vi "STAT 2 Stroker Decode Analog Data.vi"(0 "Received(T)":bool=TRUE, 7 "Controller SATT 2":T2 {"Tension Sub 2"."sys register" format="%04x"; "Tension Sub 1"."sys register" format="%04x"; "PSU"."sys register" format="%04x"; "solonoid"."valve status" format="%02x"; "solonoid"."sys register" format="%04x"; "pressure 2"."sys register" format="%04x"; "pressure 1"."sys register" format="%04x"; "Controller local"."High G monitoring" format="%02x"; "Controller local"."NA" format="%02x"; "Controller local"."GPIO values" format="%02x"; "Controller local"."Relay status" format="%02x"; "Controller local"."sys register" format="%04x"}, 11 "error in (no error)":errorcluster) -> (6 "Tool analog value":dbl[](array[numeric]), 8 "Analog for digital calc":T1, 10 "Tool analog index":u16[](array[numeric]), 14 "Solenoid position":dbl, 15 "error out":errorcluster)   [LabVIEW 2011]
uses:
  High level/Variable List Stroker Analog.ctl
  Analog values for digital calculations.ctl
  LEINmaster/Nodes/Controller local stat2.ctl
  LEINmaster/Nodes/pressure stat2.ctl
  LEINmaster/Nodes/solonoid stat2.ctl
  Stat def/Stroker system stat2.ctl
  LEINmaster/Nodes/PSU stat2.ctl
  LEINmaster/Nodes/tensionsub stat2.ctl
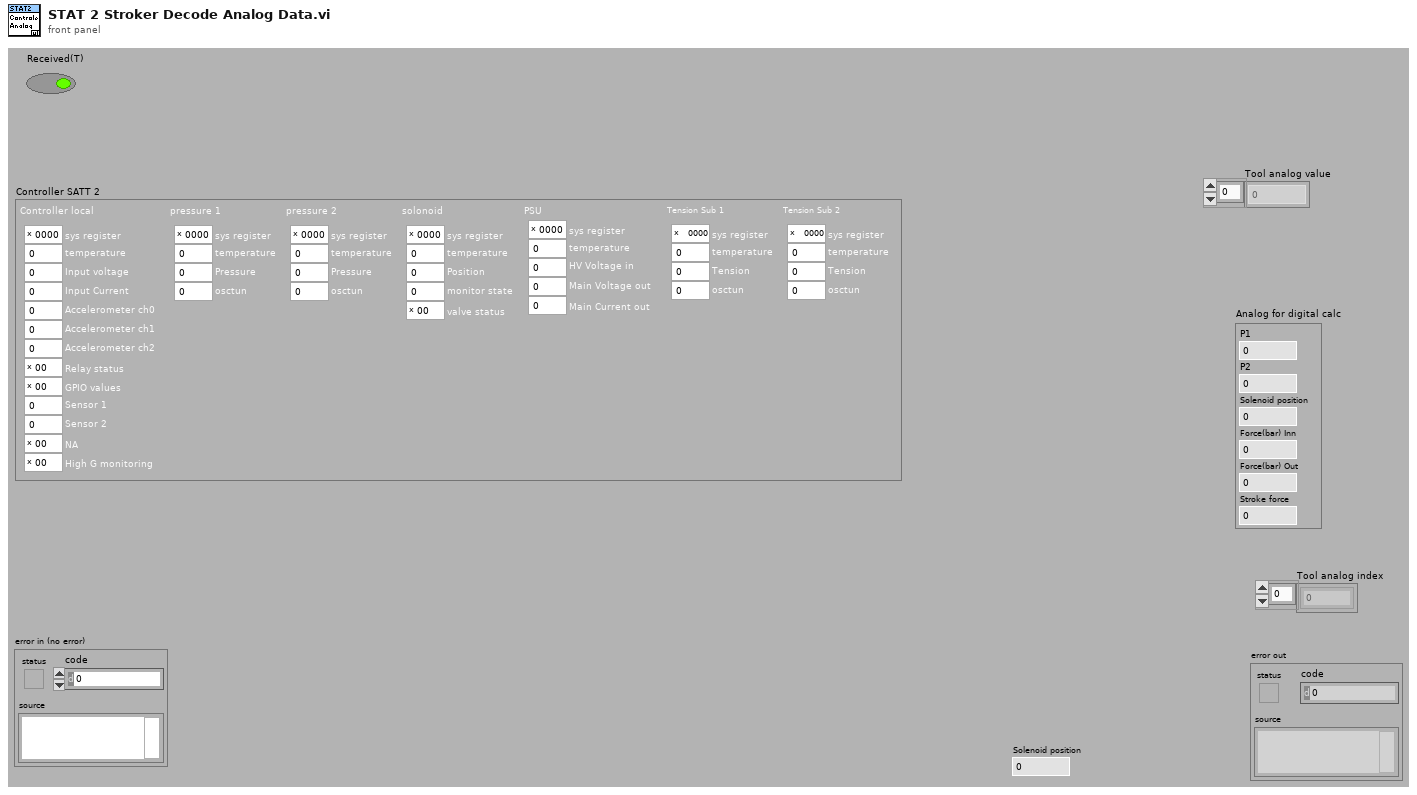
[diagram p1: front panel]
types:
  T1 = typedef "Analog values for digital calculations.ctl" = cluster{"P1":dbl, "P2":dbl, "Solenoid position":dbl, "Force(bar) Inn":dbl, "Force(bar) Out":dbl, "Stroke force":dbl}
  T2 = typedef "Stroker system stat2.ctl" = cluster{"Controller local":T3, "pressure 1":T4, "pressure 2":T4, "solonoid":T5, "PSU":T6, "Tension Sub 1":T7, "Tension Sub 2":T7}
  T3 = typedef "Controller local stat2.ctl" = cluster{"sys register":u16, "temperature":u16, "Input voltage":u16, "Input Current":u16, "Accelerometer ch0":u16, "Accelerometer ch1":u16, "Accelerometer ch2":u16, "Relay status":u8, "GPIO values":u8, "Sensor 1":i32, "Sensor 2":i32, "NA":u8, "High G monitoring":u8}
  T4 = typedef "pressure stat2.ctl" = cluster{"sys register":u16, "temperature":u16, "Pressure":u16, "osctun":u8}
  T5 = typedef "solonoid stat2.ctl" = cluster{"sys register":u16, "temperature":u16, "Position":i16, "monitor state":u8, "valve status":u8}
  T6 = typedef "PSU stat2.ctl" = cluster{"sys register":u16, "temperature":u16, "HV Voltage in":u16, "Main Voltage out":u16, "Main Current out":u16}
  T7 = typedef "tensionsub stat2.ctl" = cluster{"sys register":u16, "temperature":u16, "Tension":i16, "osctun":u8}
  T8 = typedef "Variable List Stroker Analog.ctl" = enum16{"Tool max Temperature", "Solenoid Temp", "Tool supply Voltage", "Tool (Controller) Current", "Tool Acceleration X", "Tool Acceleration Y", "Tool Acceleration Z", "Controller Temp", "Tool Acceleration Sum", "Tool Inclination", "Tool Rotation", "Tool Stroke Extension", "Tool GP Sensor 1", "Tool GP Sensor 2", "Tool (Pressure 1) Temp", "Tool Pressure 1", "Tool (Pressure 2) Temp", "Tool Pressure 2", "Do not use (SIF)", "Do not use (SOF)", "Stroke Force", "PSU Temp", "Head Voltage", "PSU Main Voltage out", "PSU Main Current out", "Upper Tension Sub Temp", "Tool Upper Tension Sub", "Lower Tension Sub Temp", "Tool Lower Tension Sub"}
  T9 = typedef "Options  All pages and custom.ctl" = cluster{"P 1 (App)":T10, "P 2":T11, "P 3":T12, "P 4":T14, "P 5":T18, "P 6 (Err)":T19, "P 7 (Expert)":T20, "C 1":T22, "C 2":T23}
  T10 = typedef "Options Page 1 (App).ctl" = cluster{"Result files":path, "PCP Interface":string, "Stroker Interface":string, "Tractor Interface":string, "Audible Alarm":bool, "Force alarm on Technical":bool, "Force alarm on HH":bool, "Force alarm on LL":bool, "Force alarm on H":bool, "Force alarm on L":bool}
  T11 = typedef "Options Page 2.ctl" = cluster{"Solenoid & Relay latching time":u16, "Tractor relay 1":dbl, "Tractor relay 2":dbl, "Tractor Solenoid limit":dbl}
  T12 = typedef "Options Page 3.ctl" = cluster{"Min resistance":dbl, "Max resistance":dbl, "PCP/PSU range":T13, "Max voltage jump":dbl, "Maximum resistance change":dbl, "Start Telemetry Voltage":dbl, "Start Telemetry Timeout":dbl, "Start Motor Voltage":dbl, "Stop Motor Voltage":dbl, "Pass Mode Warning Voltage":dbl, "Samples to average":i32}
  T13 = typedef "PCP type List.ctl" = enum16{"0 - 350V", "0 - 450V", "0 - 600V"}
  T14 = typedef "Options Page 4.ctl" = cluster{"Solenoid & Relay latching time":u16, "Stroker relay 1":dbl, "Stroker Relay 2":dbl, "Stroker Solenoid limit":dbl, "Force det.":T15, "Stroke force lim.":dbl, "Pressure SLIPS":dbl, "Tacometer puls":dbl, "Relay Voltage Limit":dbl, "Default anchor behavior":T16, "Default stroker behavior":T17, "Default stroker force limit (tonne)":dbl}
  T15 = typedef "Stroke force selector.ctl" = enum16{"Stroke in = node 1", "Strok out = node 1"}
  T16 = typedef "Default anchor behavior.ctl" = enum16{"Do nothing", "Set Anchor", "Release Anchor"}
  T17 = typedef "Default stroker behavior.ctl" = enum16{"Do nothing", "Stop", "Go Out", "Go In"}
  T18 = typedef "Options Page 5.ctl" = cluster{"Solenoid & Relay latching time":u16, "Driller relay 1":dbl, "Driller Relay 2":dbl, "Driller  Solenoid limit":dbl}
  T19 = typedef "Options Page 6 (Err).ctl" = cluster{"Error and event files":path}
  T20 = typedef "Options Page 7 (Expert).ctl" = cluster{"Show Debug":bool, "Log debug messages":bool, "Aditional debug messages":bool, "enumCANCOM":bool, "AutoLogOn":bool, "Buffer size":i32, "Modem sim":T21, "Modem baud":u16, "Upd regular data":bool, "Show Simulator":bool}
  T21 = typedef "Modem simulation setup.ctl" = cluster{"Modem dealay sim":bool, "Sim baud Tx":u16, "Bit Error fraction Tx":dbl, "Sim baud Rx":u16, "Bit Error fraction Rx":dbl}
  T22 = typedef "Options Custom 1.ctl" = cluster{"Placeholder":bool}
  T23 = typedef "Options Custom 2.ctl" = cluster{"Placeholder":bool}
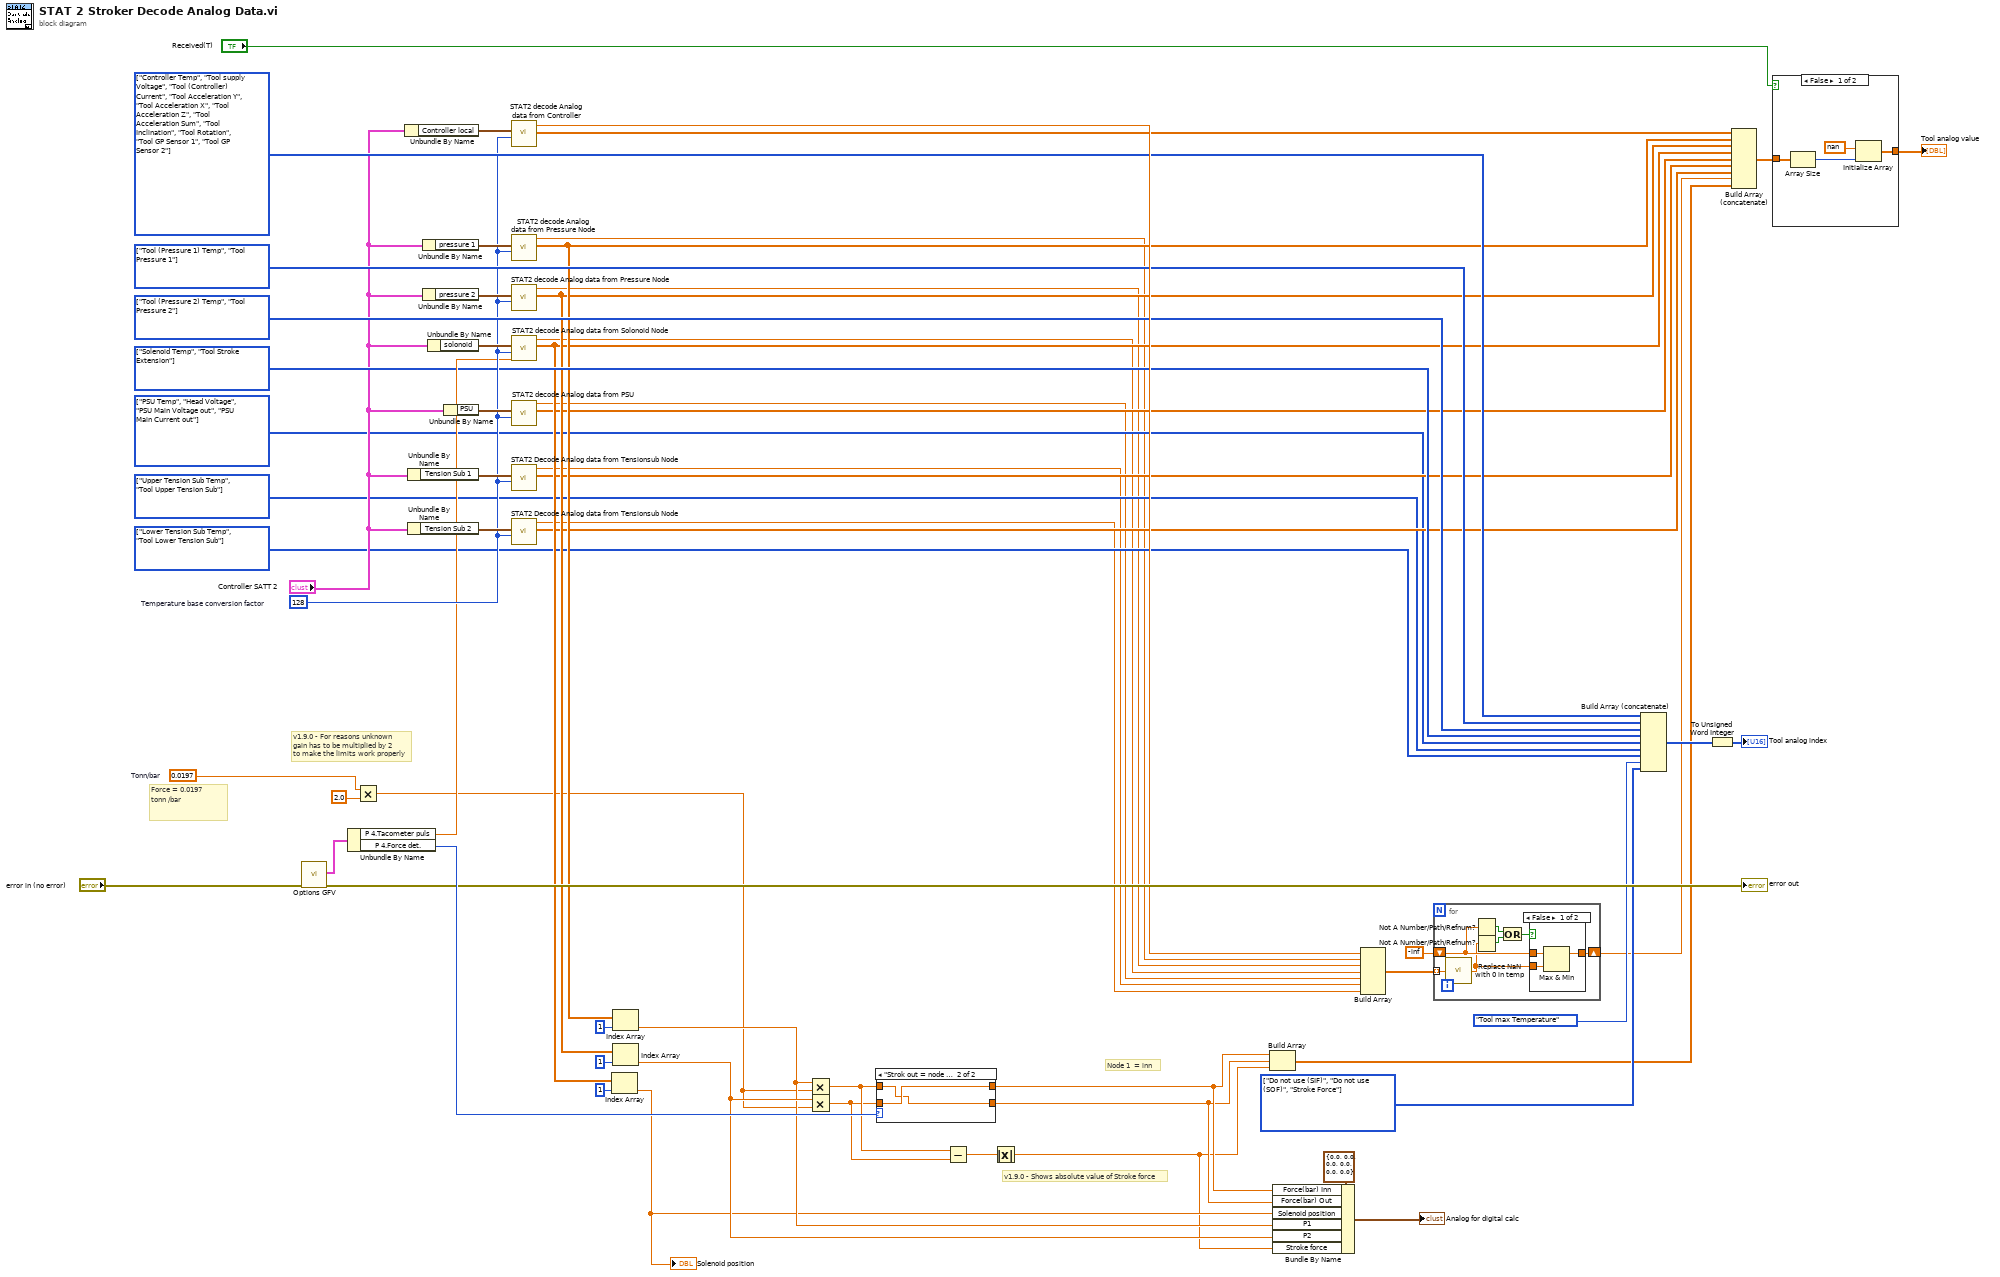
[diagram p0: block diagram]
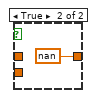
[diagram p3: hidden frame]
diagram:
  w11 = T8[] [enum."Lower Tension Sub Temp", enum."Tool Lower Tension Sub"] items=["Tool max Temperature", "Solenoid Temp", "Tool supply Voltage", "Tool (Controller) Current", "Tool Acceleration X", "Tool Acceleration Y", "Tool Acceleration Z", "Controller Temp", "Tool Acceleration Sum", "Tool Inclination", "Tool Rotation", "Tool Stroke Extension", "Tool GP Sensor 1", "Tool GP Sensor 2", "Tool (Pressure 1) Temp", "Tool Pressure 1", "Tool (Pressure 2) Temp", "Tool Pressure 2", "Do not use (SIF)", "Do not use (SOF)", "Stroke Force", "PSU Temp", "Head Voltage", "PSU Main Voltage out", "PSU Main Current out", "Upper Tension Sub Temp", "Tool Upper Tension Sub", "Lower Tension Sub Temp", "Tool Lower Tension Sub"] ("array")
  w12 = T8[] [enum."Upper Tension Sub Temp", enum."Tool Upper Tension Sub"] items=["Tool max Temperature", "Solenoid Temp", "Tool supply Voltage", "Tool (Controller) Current", "Tool Acceleration X", "Tool Acceleration Y", "Tool Acceleration Z", "Controller Temp", "Tool Acceleration Sum", "Tool Inclination", "Tool Rotation", "Tool Stroke Extension", "Tool GP Sensor 1", "Tool GP Sensor 2", "Tool (Pressure 1) Temp", "Tool Pressure 1", "Tool (Pressure 2) Temp", "Tool Pressure 2", "Do not use (SIF)", "Do not use (SOF)", "Stroke Force", "PSU Temp", "Head Voltage", "PSU Main Voltage out", "PSU Main Current out", "Upper Tension Sub Temp", "Tool Upper Tension Sub", "Lower Tension Sub Temp", "Tool Lower Tension Sub"] ("array")
  w13 = T8[] [enum."PSU Temp", enum."Head Voltage", enum."PSU Main Voltage out", enum."PSU Main Current out"] items=["Tool max Temperature", "Solenoid Temp", "Tool supply Voltage", "Tool (Controller) Current", "Tool Acceleration X", "Tool Acceleration Y", "Tool Acceleration Z", "Controller Temp", "Tool Acceleration Sum", "Tool Inclination", "Tool Rotation", "Tool Stroke Extension", "Tool GP Sensor 1", "Tool GP Sensor 2", "Tool (Pressure 1) Temp", "Tool Pressure 1", "Tool (Pressure 2) Temp", "Tool Pressure 2", "Do not use (SIF)", "Do not use (SOF)", "Stroke Force", "PSU Temp", "Head Voltage", "PSU Main Voltage out", "PSU Main Current out", "Upper Tension Sub Temp", "Tool Upper Tension Sub", "Lower Tension Sub Temp", "Tool Lower Tension Sub"]
  w24 = T8[] [enum."Solenoid Temp", enum."Tool Stroke Extension"] items=["Tool max Temperature", "Solenoid Temp", "Tool supply Voltage", "Tool (Controller) Current", "Tool Acceleration X", "Tool Acceleration Y", "Tool Acceleration Z", "Controller Temp", "Tool Acceleration Sum", "Tool Inclination", "Tool Rotation", "Tool Stroke Extension", "Tool GP Sensor 1", "Tool GP Sensor 2", "Tool (Pressure 1) Temp", "Tool Pressure 1", "Tool (Pressure 2) Temp", "Tool Pressure 2", "Do not use (SIF)", "Do not use (SOF)", "Stroke Force", "PSU Temp", "Head Voltage", "PSU Main Voltage out", "PSU Main Current out", "Upper Tension Sub Temp", "Tool Upper Tension Sub", "Lower Tension Sub Temp", "Tool Lower Tension Sub"]
  w30 = T8[] [enum."Tool (Pressure 2) Temp", enum."Tool Pressure 2"] items=["Tool max Temperature", "Solenoid Temp", "Tool supply Voltage", "Tool (Controller) Current", "Tool Acceleration X", "Tool Acceleration Y", "Tool Acceleration Z", "Controller Temp", "Tool Acceleration Sum", "Tool Inclination", "Tool Rotation", "Tool Stroke Extension", "Tool GP Sensor 1", "Tool GP Sensor 2", "Tool (Pressure 1) Temp", "Tool Pressure 1", "Tool (Pressure 2) Temp", "Tool Pressure 2", "Do not use (SIF)", "Do not use (SOF)", "Stroke Force", "PSU Temp", "Head Voltage", "PSU Main Voltage out", "PSU Main Current out", "Upper Tension Sub Temp", "Tool Upper Tension Sub", "Lower Tension Sub Temp", "Tool Lower Tension Sub"]
  w31 = T8[] [enum."Tool (Pressure 1) Temp", enum."Tool Pressure 1"] items=["Tool max Temperature", "Solenoid Temp", "Tool supply Voltage", "Tool (Controller) Current", "Tool Acceleration X", "Tool Acceleration Y", "Tool Acceleration Z", "Controller Temp", "Tool Acceleration Sum", "Tool Inclination", "Tool Rotation", "Tool Stroke Extension", "Tool GP Sensor 1", "Tool GP Sensor 2", "Tool (Pressure 1) Temp", "Tool Pressure 1", "Tool (Pressure 2) Temp", "Tool Pressure 2", "Do not use (SIF)", "Do not use (SOF)", "Stroke Force", "PSU Temp", "Head Voltage", "PSU Main Voltage out", "PSU Main Current out", "Upper Tension Sub Temp", "Tool Upper Tension Sub", "Lower Tension Sub Temp", "Tool Lower Tension Sub"]
  w32 = T8[] [enum."Controller Temp", enum."Tool supply Voltage", enum."Tool (Controller) Current", enum."Tool Acceleration Y", enum."Tool Acceleration X", enum."Tool Acceleration Z", enum."Tool Acceleration Sum", enum."Tool Inclination", enum."Tool Rotation", enum."Tool GP Sensor 1", enum."Tool GP Sensor 2"] items=["Tool max Temperature", "Solenoid Temp", "Tool supply Voltage", "Tool (Controller) Current", "Tool Acceleration X", "Tool Acceleration Y", "Tool Acceleration Z", "Controller Temp", "Tool Acceleration Sum", "Tool Inclination", "Tool Rotation", "Tool Stroke Extension", "Tool GP Sensor 1", "Tool GP Sensor 2", "Tool (Pressure 1) Temp", "Tool Pressure 1", "Tool (Pressure 2) Temp", "Tool Pressure 2", "Do not use (SIF)", "Do not use (SOF)", "Stroke Force", "PSU Temp", "Head Voltage", "PSU Main Voltage out", "PSU Main Current out", "Upper Tension Sub Temp", "Tool Upper Tension Sub", "Lower Tension Sub Temp", "Tool Lower Tension Sub"]
  w3 = 0.0197  # Tonn/bar
  w33 = T8[] [enum."Do not use (SIF)", enum."Do not use (SOF)", enum."Stroke Force"] items=["Tool max Temperature", "Solenoid Temp", "Tool supply Voltage", "Tool (Controller) Current", "Tool Acceleration X", "Tool Acceleration Y", "Tool Acceleration Z", "Controller Temp", "Tool Acceleration Sum", "Tool Inclination", "Tool Rotation", "Tool Stroke Extension", "Tool GP Sensor 1", "Tool GP Sensor 2", "Tool (Pressure 1) Temp", "Tool Pressure 1", "Tool (Pressure 2) Temp", "Tool Pressure 2", "Do not use (SIF)", "Do not use (SOF)", "Stroke Force", "PSU Temp", "Head Voltage", "PSU Main Voltage out", "PSU Main Current out", "Upper Tension Sub Temp", "Tool Upper Tension Sub", "Lower Tension Sub Temp", "Tool Lower Tension Sub"]
  w28 = u16 128  # Temperature base conversion factor
  # "v1.9.0 - For reasons unknown \ngain has to be multiplied by 2\nto make the limits work properly"
  # "v1.9.0 - Shows absolute value of Stroke force"
  # "Node 1  = inn"
  # "Force = 0.0197 tonn /bar"
  n1 = call "Options GFV.vi"("error in (no error)"="error in (no error)") -> ("Options"=w45:T9, "error out"=→"error out":errorcluster)  [unwired: 16 in, 1 out]
  n2 = Unbundle By Name(w45) -> ("P 4.Tacometer puls"=w27:dbl, "P 4.Force det."=w54:T15)
  n3 = Multiply(x=w3, y=2.0) -> (x*y=w1:dbl)
  n4 = Unbundle By Name("Controller SATT 2") -> ("Controller local"=w43:T3)
  n5 = Unbundle By Name("Controller SATT 2") -> ("Tension Sub 1"=w41:T7)
  n6 = Unbundle By Name("Controller SATT 2") -> ("Tension Sub 2"=w34:T7)
  n7 = Unbundle By Name("Controller SATT 2") -> ("pressure 1"=w40:T4)
  n8 = Unbundle By Name("Controller SATT 2") -> ("pressure 2"=w39:T4)
  n9 = Unbundle By Name("Controller SATT 2") -> ("solonoid"=w29:T5)
  n10 = Unbundle By Name("Controller SATT 2") -> ("PSU"=w42:T6)
  n11 = call "STAT2 decode Analog data from Controller.vi"("Temperature base conversion factor"=w28, "Controller local"=w43) -> ("Controller analog data"=w23:dbl[], "Temperature"=w46:dbl)  [unwired: 8 in]
  n12 = call "STAT2 decode Analog data from Pressure Node.vi"("Temperature base conversion factor"=w28, "Pressure"=w40) -> ("Node Analog value"=w22:dbl[], "Temperature"=w10:dbl)  [unwired: 8 in]
  n13 = call "STAT2 decode Analog data from Pressure Node.vi"("Temperature base conversion factor"=w28, "Pressure"=w39) -> ("Node Analog value"=w21:dbl[], "Temperature"=w9:dbl)  [unwired: 8 in]
  n14 = call "STAT2 decode Analog data from Solonoid Node.vi"(8:w27, "Temperature base conversion factor"=w28, "Solonoid"=w29) -> ("Node Analog value"=w20:dbl[], "Temperature"=w8:dbl)  [unwired: 7 in]
  n15 = call "STAT2 decode Analog data from PSU.vi"("Temperature base conversion factor"=w28, "PSU"=w42) -> ("Node Analog value"=w19:dbl[], "Temperature"=w7:dbl)  [unwired: 8 in]
  n16 = call "STAT2 Decode Analog data from Tensionsub Node.vi"("Temperature base conversion factor"=w28, "Tension Sub"=w41) -> ("Node Analog value"=w18:dbl[], "Temperature"=w6:dbl)  [unwired: 8 in]
  n17 = call "STAT2 Decode Analog data from Tensionsub Node.vi"("Temperature base conversion factor"=w28, "Tension Sub"=w34) -> ("Node Analog value"=w17:dbl[], "Temperature"=w5:dbl)  [unwired: 8 in]
  n18 = Index Array(array=w20, index=1) -> (element=w25:dbl)
  "Solenoid position" <- w25
  n19 = Index Array(array=w22, index=1) -> (element=w35:dbl)
  n20 = Index Array(array=w21, index=1) -> (element=w37:dbl)
  n21 = Multiply(x=w35, y=w1) -> (x*y=w50:dbl)
  n22 = Multiply(x=w37, y=w1) -> (x*y=w49:dbl)
  n23 = case shown="\"Strok out = node 1\"" w54 {
    tunnel: w50 -> [w65 w66]
    tunnel: w49 -> [w64 w67]
    tunnel: [w65 w67] -> w52
    tunnel: [w64 w66] -> w51
    frame "Stroke in = node 1", Default {
    }
    frame "Strok out = node 1" {
    }
  }
  n24 = Subtract(x=w50, y=w49) -> (x-y=w44:dbl)
  n25 = Absolute Value(x=w44) -> (abs(x)=w4:dbl)
  n26 = Build Array(w52, w51, w4) -> (w15:dbl[])
  n27 = Bundle By Name(cluster=T1 {"P1"=0.0, "P2"=0.0, "Solenoid position"=0.0, "Force(bar) Inn"=0.0, "Force(bar) Out"=0.0, "Stroke force"=0.0} ("Analog for digital calc"), "Force(bar) Inn"=w52, "Force(bar) Out"=w51, "Solenoid position"=w25, "P1"=w35, "P2"=w37, "Stroke force"=w4) -> (→"Analog for digital calc":T1)
  n28 = Build Array(w46, w10, w9, w8, w7, w6, w5) -> (w59:dbl[])
  n29 = for {
    tunnel: w59 -> [w69] mode=indexing
    shift-right: [w74] -> w16
    shift-left: -inf -> [w73]
    n30 = call "Replace NaN with 0 in temp.vi"("Temperature in"=w69) -> ("Temperature out"=w68:dbl)  [unwired: 14 in]
    n31 = Not A Number/Path/Refnum?(number/path/refnum=w73) -> (NaN/Path/Refnum?=w71:bool)
    n32 = Not A Number/Path/Refnum?(number/path/refnum=w68) -> (NaN/Path/Refnum?=w72:bool)
    n33 = Or(x=w71, y=w72) -> (x .or. y?=w70:bool)
    n34 = case shown="False" w70 {
      tunnel: [w77 nan] -> w74
      tunnel: w73 -> [w76 _]
      tunnel: w68 -> [w75 _]
      frame False {
        n35 = Max & Min(x=w76, y=w75) -> (max(x,y)=w77:dbl)  [unwired: 1 out]
      }
      frame True {
      }
    }
  }
  n36 = Build Array (concatenate)(w32, w31, w30, w24, w13, w12, w11, Variable_List_Stroker_Analog."Tool max Temperature" ("Action"), w33) -> (w63:T8[])
  n37 = To Unsigned Word Integer(number=w63) -> (unsigned 16bit integer=→"Tool analog index":u16[])
  n38 = Build Array (concatenate)(w23, w22, w21, w20, w19, w18, w17, w16, w15) -> (w60:dbl[])
  n39 = case shown="False" "Received(T)" {
    tunnel: [w79 w83] -> w61
    tunnel: w60 -> [w82 w83]
    frame False {
      n40 = Array Size(array=w82) -> (size(s)=w81:i32)
      n41 = Initialize Array(nan ("element"), w81) -> (w79:dbl[])
    }
    frame True {
    }
  }
  "Tool analog value" <- w61
